vi "getStatusMoving.vi"(8 "error in":errorcluster, 9 "status moving in":bool=TRUE, 10 "axis in":u8, 11 "connection ID":refnum<k5>) -> (0 "error out":errorcluster, 1 "status moving out":bool=TRUE, 2 "axis out":u8, 3 "connection ID":refnum<k5>)   [LabVIEW 2016]
panel:
  in  "Get Command":string="com.attocube.amc.status.getStatusMoving"
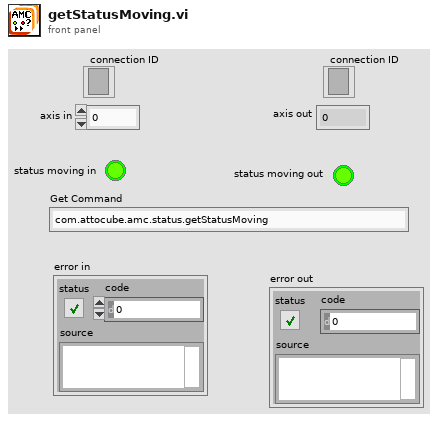
[diagram p1: front panel]
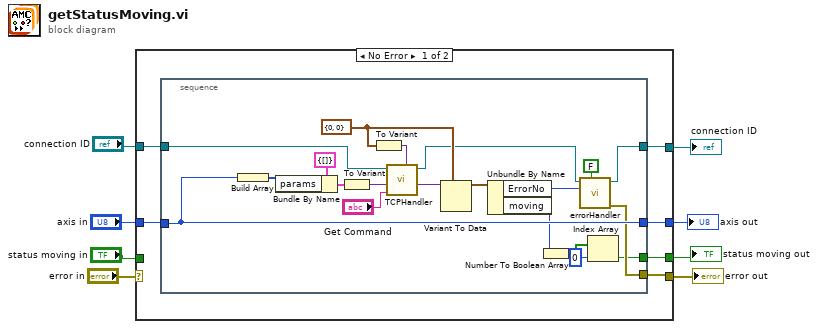
[diagram p0: block diagram]
diagram:
  n1 = case shown="No Error" "error in" {
    selector: "error in" -> [_ w36]
    tunnel: "axis in" -> [w14 w38]
    tunnel: [w9 w36] -> w7
    tunnel: [w11 w38] -> w6
    tunnel: [w10 w37] -> w5
    tunnel: [w12 w35] -> w4
    tunnel: "connection ID" -> [w13 w35]
    tunnel: "status moving in" -> [_ w37]
    frame No Error {
      n2 = stacked-sequence {
        tunnel: [w15] -> w12
        tunnel: w13 -> [w24]
        tunnel: w14 -> [w26]
        tunnel: [w26] -> w11
        tunnel: [w25] -> w9
        tunnel: [w18] -> w10
        frame #0 {
          w22 = cluster{"ErrorNo":i32, "moving":i64} {"ErrorNo"=0, "moving"=0} ("input cluster")
          n3 = Build Array(w26) -> (w30:u8[])
          n4 = Bundle By Name(cluster=cluster{"params":i32[]} {"params"=[]} ("input cluster"), "params"=w30) -> (w31:cluster{"params":i32[]})
          n5 = To Variant(anything=w31) -> (Variant=w32:variant)
          n6 = To Variant(anything=w22) -> (Variant=w23:variant)
          n7 = call "TCPHandler.vi"("result Types"=w23, "method"="Get Command", "params"=w32, "connection ID"=w24) -> ("result"=w28:variant, "connection ID"=w16:refnum<k5>)  [unwired: 5 in, 1 out]
          n8 = Variant To Data(type=w22, Variant=w28) -> (data=w33:cluster{"ErrorNo":i32, "moving":i64})  [unwired: 1 in, 1 out]
          n9 = Unbundle By Name(w33) -> ("ErrorNo"=w34:i32, "moving"=w19:i64)
          n10 = Number To Boolean Array(number=w19) -> (Boolean array=w20:bool[])
          n11 = call "errorHandler.vi"("show popup"=FALSE, "error number"=w34, "connection ID"=w16) -> ("error out"=w25:errorcluster, "connection ID"=w15:refnum<k5>)  [unwired: 7 in]
          n12 = Index Array(array=w20, index=0) -> (element=w18:bool)
        }
      }
    }
    frame Error {
    }
  }
  "error out" <- w7
  "axis out" <- w6
  "status moving out" <- w5
  "connection ID" <- w4
